vi "BLED1112-Rx Packet parser (Get Rssi).vi"(5 "message package":u8[](array[numeric])=[0, 3, 6, 3, 0, 0, 0] format="%02x") -> (0 "message out":u8[](array[numeric])=[0, 3, 6, 3, 0, 0, 0] format="%02x", 1 "Packet OK":bool, 2 "Data Structure":T1={"Message Type (Response)"=0, "Payload length"=3, "Message class"=6, "Message ID"=3, "connection"=0, "rssi"=0} {"Message class" format="%02x"; "rssi" format="%0d"; "connection" format="%02x"; "Message ID" format="%02x"; "Message Type (Response)" format="%02x" items=["Command / Response"=0, "Event"=128]})   [LabVIEW 2015]
uses:
  Lib_Bled112 toolkit/type_def/message_type.ctl
panel:
  # "Rx Packet parser (RESPONSE GAP)"
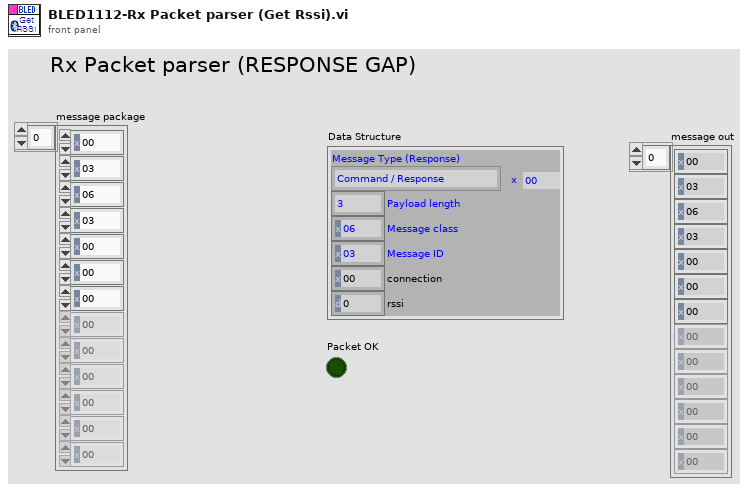
[diagram p1: front panel]
types:
  T1 = typedef "컨트롤-BLED Rx (Get RSSI).ctl" = cluster{"Message Type (Response)":T2, "Payload length":u8, "Message class":u8, "Message ID":u8, "connection":u8, "rssi":i16}
  T2 = typedef "message_type.ctl" = u8
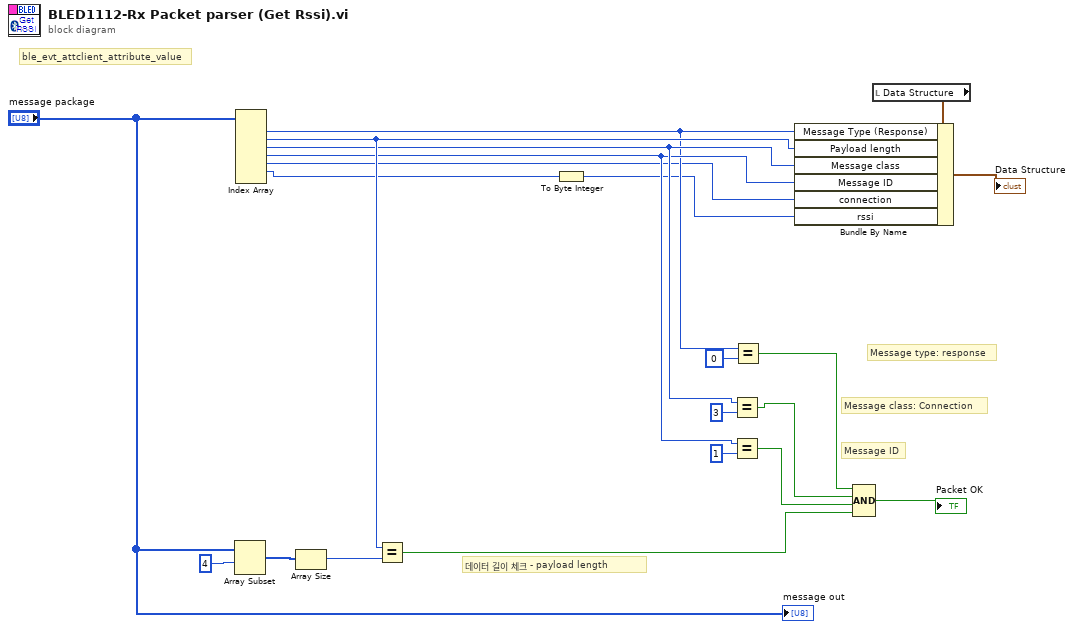
[diagram p0: block diagram]
diagram:
  # "Message type: response"
  # "Message ID"
  # "Message class: Connection"
  # "데이터 길이 체크 - payload length"
  # "ble_evt_attclient_attribute_value"
  n1 = Array Subset(array="message package", index=4 ("인덱스")) -> (w17:u8[])  [unwired: 1 in]
  n2 = Index Array(array="message package") -> (element #1=w4:u8, element #2=w19:u8, element #3=w8:u8, element #4=w7:u8, element #5=w3:u8, element #6=w2:u8)  [unwired: 7 in, 1 out]
  n3 = Array Size(array=w17) -> (size(s)=w16:i32)
  n4 = Equal?(x=w19, y=w16) -> (x = y?=w9:bool)
  n5 = To Byte Integer(number=w2) -> (8bit integer=w1:i8)
  n6 = Equal?(x=w8, y=3 ("인덱스")) -> (x = y?=w11:bool)
  n7 = Equal?(x=w7, y=1 ("인덱스")) -> (x = y?=w12:bool)
  n8 = Equal?(x=w4, y=0 ("인덱스")) -> (x = y?=w5:bool)
  n9 = Compound Arithmetic op=AND ("복합 연산")(w5, w11, w12, w9) -> (→"Packet OK":bool)
  n10 = local read "Data Structure"() -> (w21:T1)
  n11 = Bundle By Name(cluster=w21, "Message Type (Response)"=w4, "Payload length"=w19, "Message class"=w8, "Message ID"=w7, "connection"=w3, "rssi"=w1) -> (→"Data Structure":T1)
  "message out" <- "message package"
